vi "Initialize Galil IO.vi"(0 "Galil.IGalil":refnum<k7>, 1 "Command Input":string="TLA=0;ACA=150000;DCA=300000;SPA=125000;SHA;PTA=1;PAA=10000;TLB=9.8;ACB=250000;DCB=500000;SPB=200000;SHB;PTB=1;DPB=", 5 "Initial Encoder Counts":string="0" caption="Enter number in encoder counts, 0 is middle, -650000 fully entended; 650000 fully retracted") -> (2 "address":string="192.168.1.10", 3 "timeout_ms":i32=500, 4 "Error - Query Connection":errorcluster, 6 "Reference Out":refnum<k7>, 7 "addresses":variant, 8 "Error - Establish Connection":errorcluster, 9 "Error Out":errorcluster)   [LabVIEW 2011]
uses:
  _GlobalVariables&Libraries/ATV Program Global Variables 2.vi
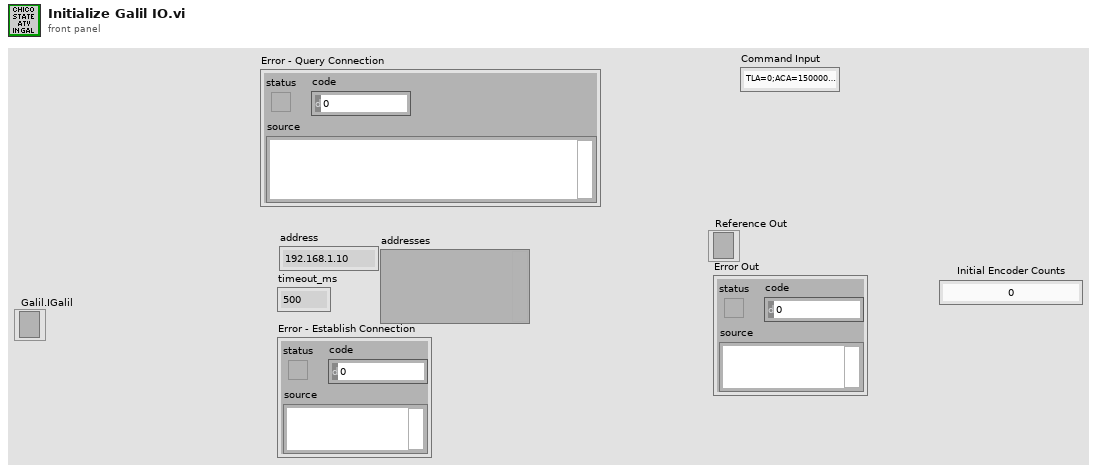
[diagram p1: front panel]
types:
  T1 = cluster{"Drive Value Output String":string, "Steer Value Output String":string, "Error Out":errorcluster, "Initial Encoder Counts":string, "Disable Galil Terminal":bool, "Command Input":string}
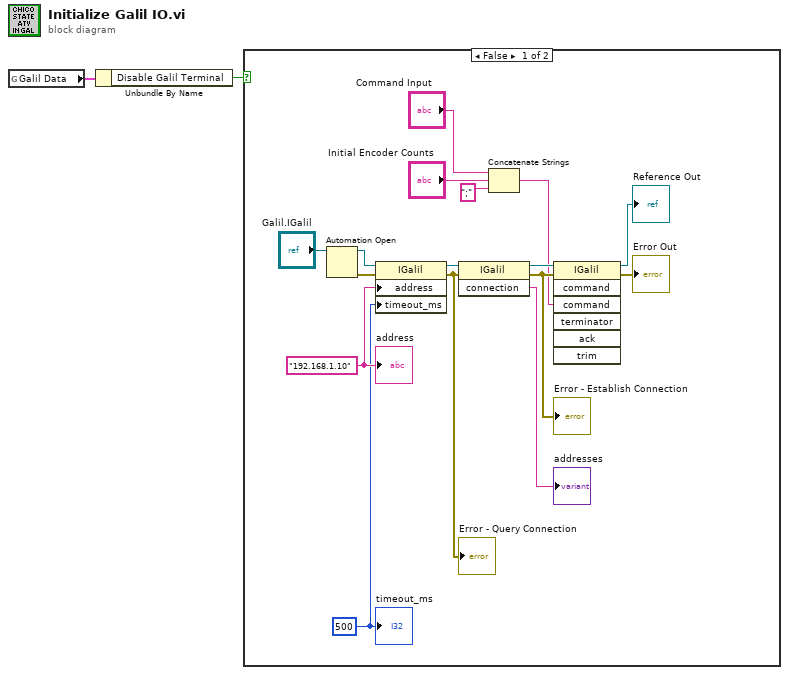
[diagram p0: block diagram]
diagram:
  n1 = global read "ATV Program Global Variables 2.vi" "Galil Data"() -> (w2:T1)
  n2 = Unbundle By Name(w2) -> ("Disable Galil Terminal"=w1:bool)
  n3 = case shown="False" w1 {
    frame False {
      w7 = 500 ("timeout_ms")
      w8 = "192.168.1.10" ("address")
      n4 = Automation Open(Automation Refnum="Galil.IGalil") -> (Automation Refnum=w15:refnum<k7>, error out=w14:errorcluster)  [unwired: 3 in]
      n5 = property class="IGalil"(reference=w15, error in=w14, "address"=w8, "timeout_ms"=w7) -> (reference out=w12:refnum<k7>, error out=w13:errorcluster)
      "Error - Query Connection" <- w13
      n6 = invoke class="IGalil" method="connection"(reference=w12, error in=w13) -> (reference out=w9:refnum<k7>, error out=w10:errorcluster, "connection"=→"addresses":string)  [unwired: 1 in]
      "Error - Establish Connection" <- w10
      n7 = Concatenate Strings("Command Input", "Initial Encoder Counts", ";" ("string")) -> (w3:string)
      n8 = invoke class="IGalil" method="command"(reference=w9, error in=w10, "command"=w3) -> (reference out=→"Reference Out":refnum<k7>, error out=→"Error Out":errorcluster)  [unwired: 4 in, 5 out]
      "address" <- w8
      "timeout_ms" <- w7
    }
    frame True {
    }
  }
